vi "Ke2400 Measurement.vi"(8 "error in (no error)":errorcluster, 11 "VISA in":refnum<visa-resource-name>) -> (0 "error out":errorcluster, 1 "Voltage(V)":string, 2 "uA":string, 3 "VISA Out":refnum<visa-resource-name>, 4 "Res(Ohm)":string)   [LabVIEW 2012]
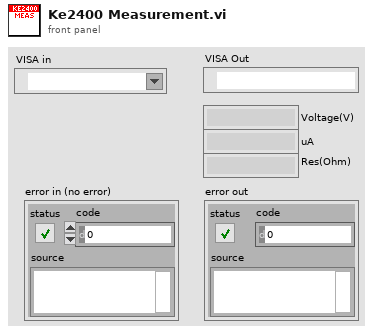
[diagram p1: front panel]
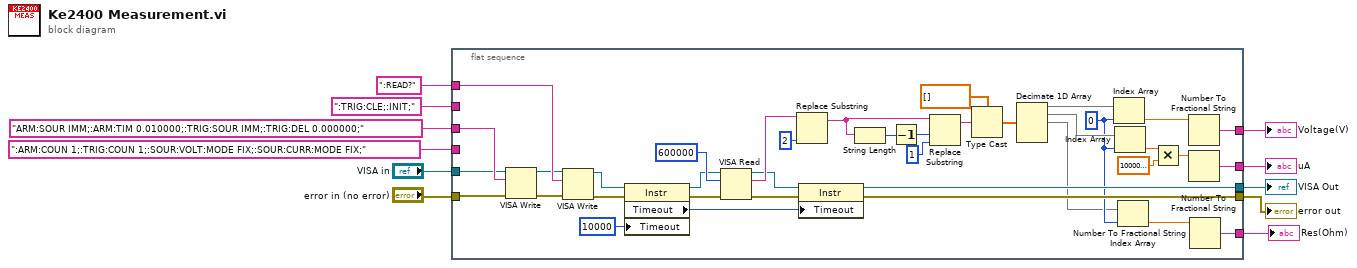
[diagram p0: block diagram]
diagram:
  n1 = flat-sequence {
    tunnel: [w25] -> w11
    tunnel: "VISA in" -> [w23]
    tunnel: "error in (no error)" -> [w22]
    tunnel: [w36] -> w8
    tunnel: [w28] -> w7
    tunnel: "ARM:SOUR IMM;:ARM:TIM 0.010000;:TRIG:SOUR IMM;:TRIG:DEL 0.000000;" ("resulting string") -> [w35]
    tunnel: ":TRIG:CLE;:INIT;" ("write buffer") -> [_]
    tunnel: ":READ?" ("write buffer") -> [w34]
    tunnel: ":ARM:COUN 1;:TRIG:COUN 1;:SOUR:VOLT:MODE FIX;:SOUR:CURR:MODE FIX;" ("write buffer") -> [_]
    tunnel: [w17] -> w2
    tunnel: [w13] -> w1
    frame #0 {
      w15 = 0 ("index")
      n2 = VISA Write(VISA resource name=w23, write buffer=w35, error in (no error)=w22) -> (VISA resource name out=w21:refnum<visa-resource-name>, error out=w20:errorcluster)  [unwired: 1 out]
      n3 = VISA Write(VISA resource name=w21, write buffer=w34, error in (no error)=w20) -> (VISA resource name out=w32:refnum<visa-resource-name>, error out=w33:errorcluster)  [unwired: 1 out]
      n4 = property class="Instr"(reference=w32, error in=w33, "Timeout"=u32 10000 ("General Settings:Timeout Value")) -> (reference out=w31:refnum<visa-resource-name>, error out=w30:errorcluster, "Timeout"=w27:u32)
      n5 = VISA Read(VISA resource name=w31, byte count=u32 600000, error in (no error)=w30) -> (VISA resource name out=w29:refnum<visa-resource-name>, read buffer=w38:string, error out=w26:errorcluster)  [unwired: 1 out]
      n6 = Replace Substring(2:2 ("length (len. of substring)"), 5:w38) -> (1:w46:string)  [unwired: 2 in, 1 out]
      n7 = property class="Instr"(reference=w29, error in=w26, "Timeout"=w27) -> (reference out=w28:refnum<visa-resource-name>, error out=w25:errorcluster)
      n8 = String Length(string=w46) -> (length=w42:i32)
      n9 = Decrement(x=w42) -> (x-1=w41:i32)
      n10 = Replace Substring(2:1 ("length (len. of substring)"), 3:w41, 5:w46) -> (1:w43:string)  [unwired: 1 in, 1 out]
      n11 = Type Cast(type=sgl[] [], x=w43) -> (*(type *) &x=w45:sgl[])
      n12 = Decimate 1D Array(w45) -> (w19:sgl[], w16:sgl[], w12:sgl[])  [unwired: 2 out]
      n13 = Index Array(array=w19, index=w15) -> (element=w18:sgl)
      n14 = Index Array(array=w16, index=w15) -> (element=w47:sgl)
      n15 = Index Array(array=w12, index=w15) -> (element=w14:sgl)
      n16 = Multiply(x=w47, y=sgl 1000000.0) -> (x*y=w49:sgl)
      n17 = Number To Fractional String(number=w18) -> (F-format string=w17:string)  [unwired: 3 in]
      n18 = Number To Fractional String(number=w49) -> (F-format string=w36:string)  [unwired: 3 in]
      n19 = Number To Fractional String(number=w14) -> (F-format string=w13:string)  [unwired: 3 in]
    }
  }
  "error out" <- w11
  "uA" <- w8
  "VISA Out" <- w7
  "Voltage(V)" <- w2
  "Res(Ohm)" <- w1
